vi "eth_spi.vi"() -> ()   [LabVIEW 2015]
panel:
  in  "Port":string
  in  "Write Data":string
  in  "IP Address":string
  out "error out":errorcluster
  out "String":string
  in  "Chip Select":u32
  in  "Clock Rate in kHz":u16=1000
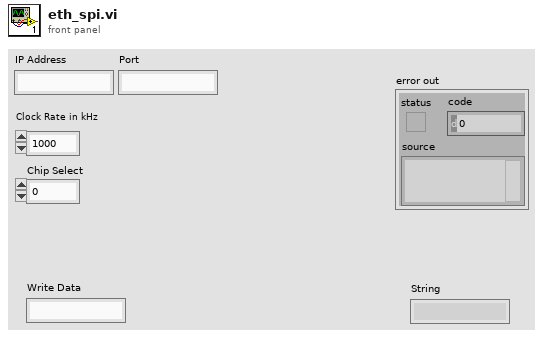
[diagram p1: front panel]
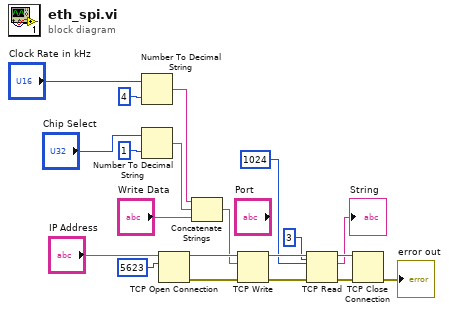
[diagram p0: block diagram]
diagram:
  n1 = Number To Decimal String(number="Clock Rate in kHz", width (-)=4) -> (decimal integer string=w9:string)
  n2 = Number To Decimal String(number="Chip Select", width (-)=1) -> (decimal integer string=w8:string)
  n3 = TCP Open Connection(address="IP Address", remote port or service name=5623) -> (connection ID=w19:refnum<k5>, error out=w14:errorcluster)  [unwired: 3 in]
  n4 = Concatenate Strings(w9, w8, "Write Data") -> (w7:string)
  n5 = TCP Write(connection ID=w19, data in=w7, error in (no error)=w14) -> (connection ID out=w18:refnum<k5>, error out=w15:errorcluster)  [unwired: 1 in, 1 out]
  n6 = TCP Read(connection ID=w18, bytes to read=1024, error in (no error)=w15, 7:3) -> (connection ID out=w16:refnum<k5>, data out=→"String":string, error out=w17:errorcluster)  [unwired: 1 in]
  n7 = TCP Close Connection(connection ID=w16, error in (no error)=w17) -> (error out=→"error out":errorcluster)  [unwired: 1 in, 1 out]
